vi "0816039.vi"() -> ()   [LabVIEW 2021]
panel:
  out "%.1f":T1={"[0]"=TRUE, "[1]"=TRUE, "[2]"=TRUE, "[3]"=FALSE, "[4]"=FALSE, "[5]"=TRUE, "[6]"=TRUE}
  out "Boolean":bool
  out "1":T1={"[0]"=TRUE, "[1]"=TRUE, "[2]"=TRUE, "[3]"=FALSE, "[4]"=FALSE, "[5]"=TRUE, "[6]"=TRUE}
  in  "Numeric":dbl=123.4
  out "10":T1={"[0]"=TRUE, "[1]"=TRUE, "[2]"=TRUE, "[3]"=FALSE, "[4]"=TRUE, "[5]"=TRUE, "[6]"=FALSE}
  out "100":T1={"[0]"=FALSE, "[1]"=FALSE, "[2]"=FALSE, "[3]"=FALSE, "[4]"=FALSE, "[5]"=TRUE, "[6]"=TRUE}
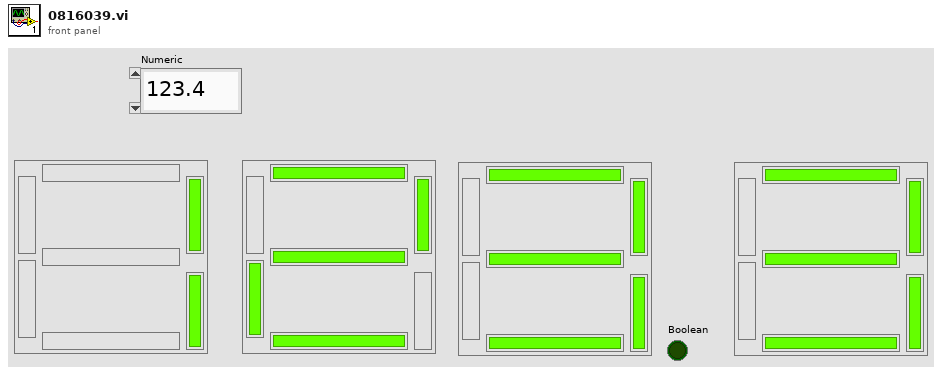
[diagram p1: front panel]
types:
  T1 = cluster{"[0]":bool, "[1]":bool, "[2]":bool, "[3]":bool, "[4]":bool, "[5]":bool, "[6]":bool}
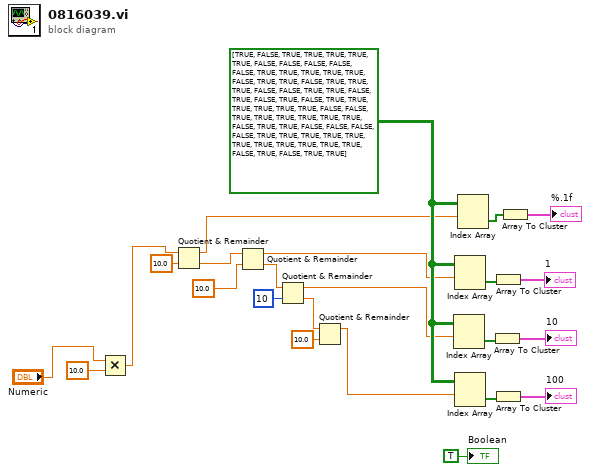
[diagram p0: block diagram]
diagram:
  w12 = bool[][] [[TRUE, FALSE, TRUE, TRUE, TRUE, TRUE, TRUE], [FALSE, FALSE, FALSE, FALSE, FALSE, TRUE, TRUE], [TRUE, TRUE, TRUE, FALSE, TRUE, TRUE, FALSE], [TRUE, TRUE, TRUE, FALSE, FALSE, TRUE, TRUE], [FALSE, TRUE, FALSE, TRUE, FALSE, TRUE, TRUE], [TRUE, TRUE, TRUE, TRUE, FALSE, FALSE, TRUE], [TRUE, TRUE, TRUE, TRUE, TRUE, FALSE, TRUE], [TRUE, FALSE, FALSE, FALSE, FALSE, TRUE, TRUE], [TRUE, TRUE, TRUE, TRUE, TRUE, TRUE, TRUE], [TRUE, TRUE, FALSE, TRUE, FALSE, TRUE, TRUE]]
  n1 = Multiply(x="Numeric", y=10.0) -> (x*y=w10:dbl)
  n2 = Quotient & Remainder(x=w10, y=10.0 ("floor(x/y)")) -> (x-y*floor(x/y)=w9:dbl, floor(x/y)=w8:dbl)
  n3 = Quotient & Remainder(x=w8, y=10.0) -> (x-y*floor(x/y)=w6:dbl, floor(x/y)=w5:dbl)
  n4 = Quotient & Remainder(x=w5, y=u32 10) -> (x-y*floor(x/y)=w4:dbl, floor(x/y)=w2:dbl)
  n5 = Quotient & Remainder(x=w2, y=10.0 ("floor(x/y)")) -> (x-y*floor(x/y)=w1:dbl)  [unwired: 1 out]
  n6 = Index Array "Index Array"(array=w12, index (row)=w4) -> (element=w21:bool[])  [unwired: 1 in]
  n7 = Index Array "Index Array"(array=w12, index (row)=w6) -> (element=w20:bool[])  [unwired: 1 in]
  n8 = Index Array "Index Array"(array=w12, index (row)=w1) -> (element=w24:bool[])  [unwired: 1 in]
  n9 = Index Array(array=w12, index (row)=w9) -> (element=w11:bool[])  [unwired: 1 in]
  n10 = Array To Cluster(array=w21) -> (cluster=→"10":T1)
  n11 = Array To Cluster(array=w20) -> (cluster=→"1":T1)
  n12 = Array To Cluster(array=w24) -> (cluster=→"100":T1)
  n13 = Array To Cluster(array=w11) -> (cluster=→"%.1f":T1)
  "Boolean" <- TRUE ("Boolean")
